vi "Set Gain.vi"(8 "error in":errorcluster, 11 "IMG_SRC in":refnum<class "IMG_SRC.lvclass">) -> (0 "error out":errorcluster, 2 "Supported?":bool, 3 "IMG_SRC out":refnum<class "IMG_SRC.lvclass">)   [LabVIEW 2018, in "IMG_SRC.lvlib" / "IMG_SRC.lvclass"]
uses:
  IMG_SRC.lvclass
  IMG_SRC.lvclass/IMG_SRC.ctl
  builds/Camera.lvlibp/Camera.lvclass
  C:/Users/Ron.Dexter.LUMINARTECH/Desktop/builds/Camera.lvlibp/Camera.lvclass
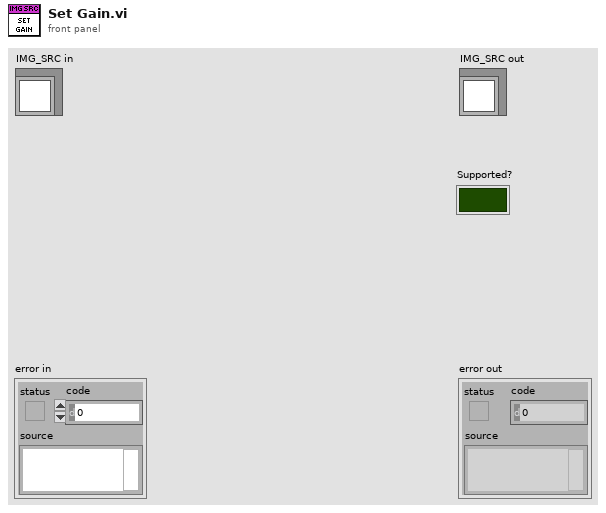
[diagram p1: front panel]
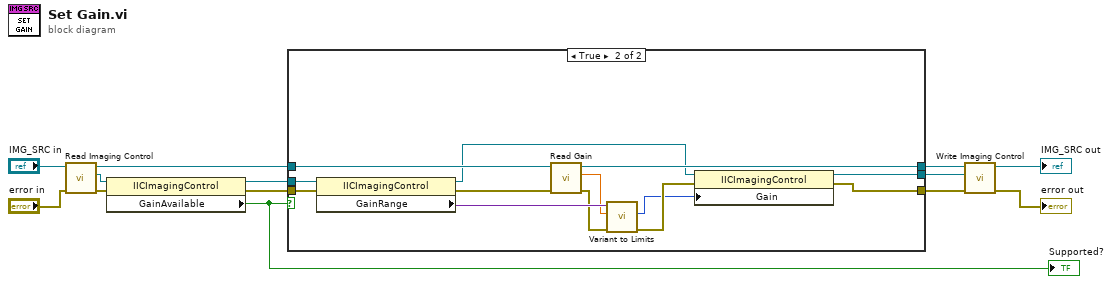
[diagram p0: block diagram]
diagram:
  n1 = call "Read Imaging Control.vi"("error in (no error)"="error in", "IMG_SRC in"="IMG_SRC in") -> ("error out"=w11:errorcluster, "Imaging Control"=w10:refnum<k7>, "IMG_SRC out"=w9:refnum<class "IMG_SRC.lvclass">)  [unwired: 7 in]
  n2 = property class="IICImagingControl"(reference=w10, error in=w11) -> (reference out=w8:refnum<k7>, error out=w7:errorcluster, "GainAvailable"=w1:bool)
  "Supported?" <- w1
  n3 = case shown="True" w1 {
    tunnel: w9 -> [w14 w26]
    tunnel: w8 -> [w15 w29]
    tunnel: w7 -> [w16 w27]
    tunnel: [w14 w25] -> w4
    tunnel: [w15 w18] -> w3
    tunnel: [w16 w17] -> w2
    frame False {
    }
    frame True {
      n4 = property class="IICImagingControl"(reference=w29, error in=w27) -> (reference out=w19:refnum<k7>, error out=w24:errorcluster, "GainRange"=w28:variant)
      n5 = call "Read Gain.vi"("error in (no error)"=w24, "Camera in"=w26) -> ("error out"=w22:errorcluster, "Gain"=w23:dbl, "Camera out"=w25:refnum<class "IMG_SRC.lvclass">)  [unwired: 7 in]
      n6 = call "Variant to Limits.vi"("error in"=w22, "Setpoint"=w23, "Variant"=w28) -> ("error out"=w21:errorcluster, "coerced setpoint"=w20:i32)  [unwired: 7 in]
      n7 = property class="IICImagingControl"(reference=w19, error in=w21, "Gain"=w20) -> (reference out=w18:refnum<k7>, error out=w17:errorcluster)
    }
  }
  n8 = call "Write Imaging Control.vi"("error in (no error)"=w2, "Imaging Control"=w3, "IMG_SRC in"=w4) -> ("error out"=→"error out":errorcluster, "IMG_SRC out"=→"IMG_SRC out":refnum<class "IMG_SRC.lvclass">)  [unwired: 7 in]
